vi "Sim_Climb.vi"(9 "StartPoseDegrees":dbl, 11 "Motor1 Dmd":dbl) -> (0 "Motor Current":dbl, 1 "At Outer Limit":bool, 2 "At Climbed Limit":bool, 3 "ClimbPositionDegrees":dbl, 4 "Voltage":dbl)   [LabVIEW 2023]
uses:
  <vilib>/Rock Robotics/WPI/ThirdParty/JAS_Junk/TrajLib/Enum/DCMOTOR_TYPES_ENUM.ctl
  <vilib>/Rock Robotics/WPI/ThirdParty/JAS_Junk/TrajLib/BatterySim_CalculateLoadedBatteryVoltage.vi
  <vilib>/Rock Robotics/WPI/ThirdParty/JAS_Junk/TrajLib/Trajectory_Library.lvlib
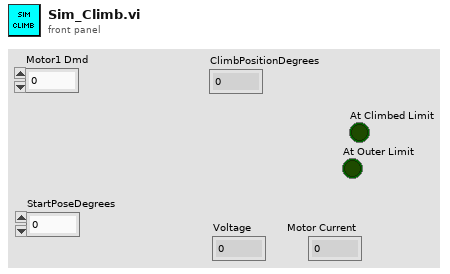
[diagram p1: front panel]
types:
  T1 = typedef "Trajectory_Library.lvlib/DCMOTOR_TYPES_ENUM.ctl" = enum16{"CIM", "AndyMark 9015", "Andy Mark RS 775 125", "Bag", "BaneBots RS 550", "BaneBots RS 775", "Falcon 500", "Mini CIM", "NEO", "NEO 550", "Romi BuiltIn", "Vex 775 Pro", "Snow Blower AM 2235A", "Bosch Seat AM 3493", "Falcon 500 FOC", "Kraken X60", "Kraken X60 FOC", "NEO Vortex"}
  T2 = typedef "Trajectory_Library.lvlib/LINEAR_SYSTEM_ID_SINGLE_JOINT_ARM_MODEL.ctl" = cluster{"DCMOTOR_TYPES":T1, "Num Motors":i32, "ArmLength_M":dbl, "massKg":dbl, "Gearing":dbl, "MOI kgm2":dbl, "Estimate MOI":bool}
  T3 = typedef "Trajectory_Library.lvlib/SINGLE_JOINT_ARM_SIM_SIMULATION_PARAMS.ctl" = cluster{"MinAngle_Rad":dbl, "MaxAngle_Rad":dbl, "Measurment StdDev":dbl, "SimulateGravity":bool}
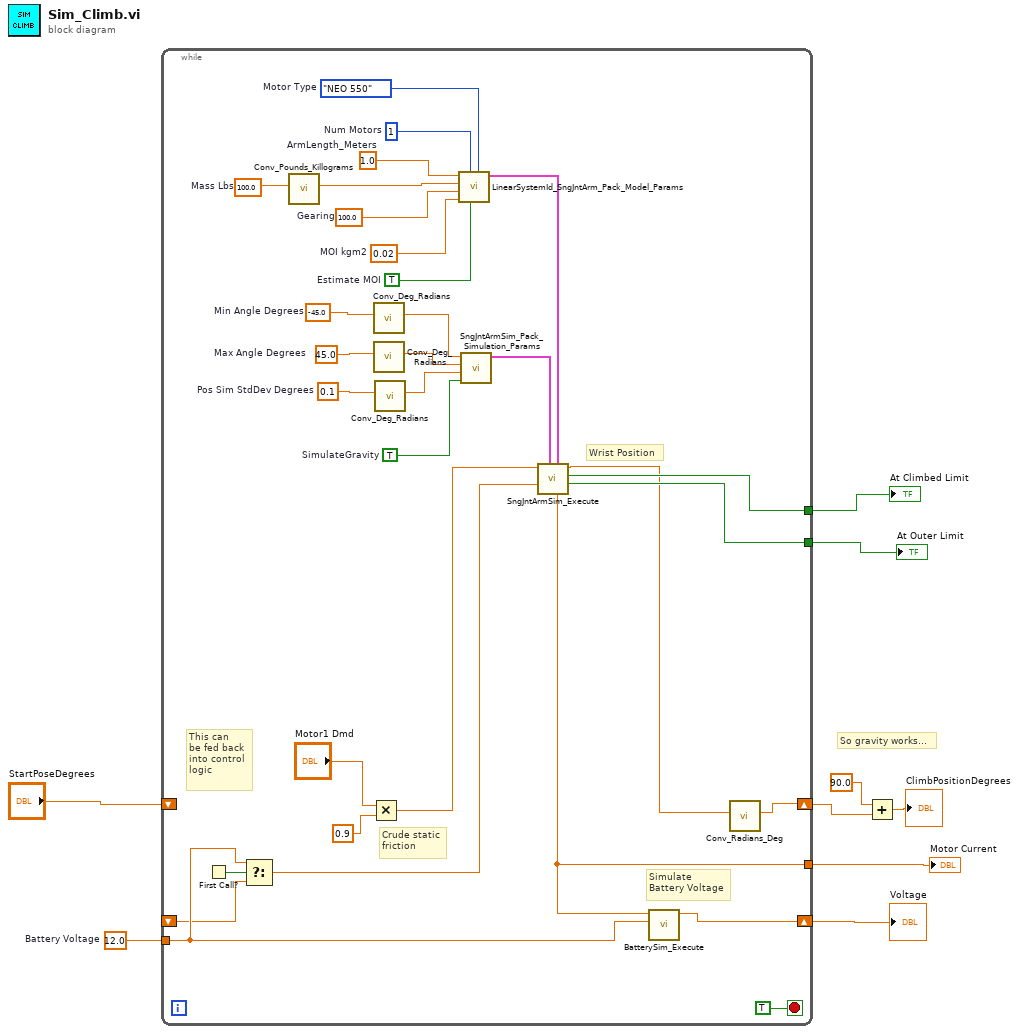
[diagram p0: block diagram]
diagram:
  w9 = 12.0  # Battery Voltage
  # "So gravity works..."
  n1 = while {
    shift-right: [w40] -> w7
    shift-left: _ -> [w36]
    shift-right: [w21] -> w3
    shift-left: "StartPoseDegrees" -> [_]
    tunnel: w9 -> [w37]
    tunnel: [w23] -> w6
    tunnel: [w22] -> w5
    tunnel: [w10] -> w4
    stop <- TRUE stop-if-true
    w28 = TRUE  # Estimate MOI
    w29 = 0.02  # MOI kgm2
    w16 = -45.0  # Min Angle Degrees
    w17 = 45.0  # Max Angle Degrees
    w18 = 0.1  # Pos Sim StdDev Degrees
    w30 = TRUE  # SimulateGravity
    w31 = 1.0  # ArmLength_Meters
    w32 = 100.0  # Gearing
    w12 = 100.0  # Mass Lbs
    w33 = 1  # Num Motors
    w34 = DCMOTOR_TYPES_ENUM."NEO 550"  # Motor Type
    # "Wrist Position"
    # "Crude static\nfriction"
    # "This can\nbe fed back\ninto control\nlogic"
    # "Simulate\nBattery Voltage"
    n2 = First Call?() -> (First Call?: T/F=w38:bool)
    n3 = Select(t=w37, s=w38, f=w36) -> (s? t:f=w19:dbl)
    n4 = call <vilib>:"Conv_Pounds_Killograms.vi"("Pounds"=w12) -> ("Killograms"=w11:dbl)  [unwired: 10 in]
    n5 = Multiply(x="Motor1 Dmd", y=0.9) -> (x*y=w24:dbl)
    n6 = call <vilib>:"Conv_Deg_Radians.vi"("Degress"=w16) -> ("Radians"=w15:dbl)  [unwired: 10 in]
    n7 = call <vilib>:"Conv_Deg_Radians.vi"("Degress"=w17) -> ("Radians"=w14:dbl)  [unwired: 10 in]
    n8 = call <vilib>:"Conv_Deg_Radians.vi"("Degress"=w18) -> ("Radians"=w13:dbl)  [unwired: 10 in]
    n9 = call <vilib>:"LinearSystemId_SngJntArm_Pack_Model_Params.vi"("DCMOTOR_TYPES"=w34, "Estimate MOI"=w28, "Num Motors"=w33, "MOI kgm2"=w29, "Gearing"=w32, "massKg"=w11, "ArmLength_M"=w31) -> ("SngJntArmSim_Model _Params"=w27:T2)  [unwired: 4 in]
    n10 = call <vilib>:"SngJntArmSim_Pack_Simulation_Params.vi"("SimulateGravity"=w30, "Pos Sim StdDev Rad"=w13, "MaxAngle_Rad"=w14, "MinAngle_Rad"=w15) -> ("SngJntArmSim_Simulation _Params"=w26:T3)  [unwired: 7 in]
    n11 = call <vilib>:"SngJntArmSim_Execute.vi"("SngJntArmSim_Model _Params"=w27, "SngJntArmSim_Simulation _Params"=w26, "Battery Volts"=w19, "Motor Dmd"=w24) -> ("AtLowLimit"=w22:bool, "At HIgh LImit"=w23:bool, "ArmAngle_Rad"=w20:dbl, "Motor Current"=w10:dbl)  [unwired: 2 in, 2 out]
    n12 = call <vilib>:"BatterySim_Execute.vi"("Nominal Battery Voltage"=w37, "Current"=w10) -> ("Voltage"=w40:dbl)  [unwired: 9 in]
    n13 = call <vilib>:"Conv_Radians_Deg.vi"("Radians"=w20) -> ("Degrees"=w21:dbl)  [unwired: 10 in]
  }
  "Voltage" <- w7
  "At Climbed Limit" <- w6
  "At Outer Limit" <- w5
  "Motor Current" <- w4
  n14 = Add(x=90.0, y=w3) -> (x+y=→"ClimbPositionDegrees":dbl)
